vi "getAllSpectraFromFolder.vi"(11 "Spectra Folder::":path) -> (2 "spectra":dbl[][][](array[numeric]) caption="spectrum\n\n\nFrequency\n\n\nColumn")   [LabVIEW 2013]
panel:
  out "All Files in Dir":path[](array[path])
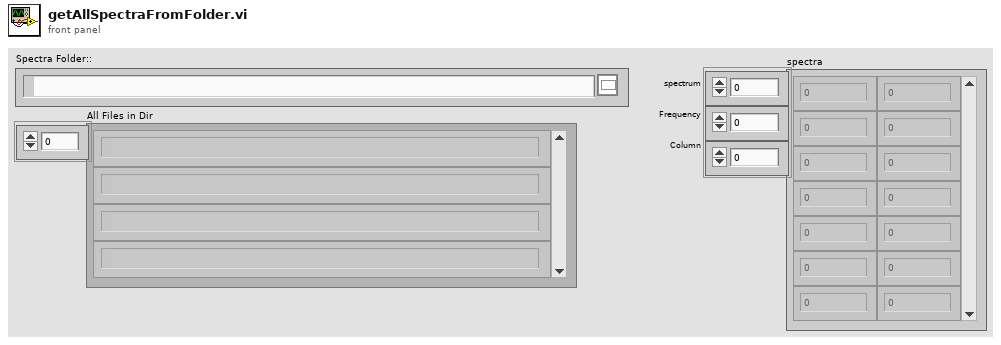
[diagram p1: front panel]
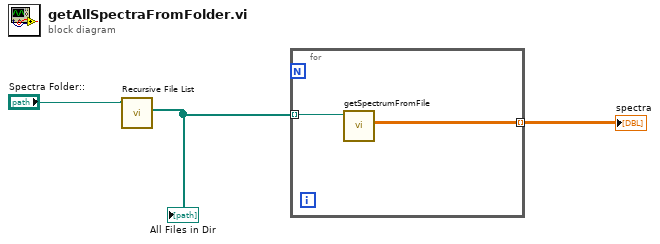
[diagram p0: block diagram]
diagram:
  n1 = call <vilib>:"Recursive File List.vi"("Folder Path"="Spectra Folder::") -> ("All Files in Dir"=w2:path[])  [unwired: 6 in, 4 out]
  "All Files in Dir" <- w2
  n2 = for {
    tunnel: w2 -> [w5] mode=indexing
    tunnel: [w4] -> w1 mode=indexing
    n3 = call "getSpectrumFromFile.vi"("File Path Control"=w5) -> ("array"=w4:dbl[][])  [unwired: 10 in]
  }
  "spectra" <- w1
